vi "_PC_Daemon_TurboPump.vi"(7 "engModeStr":refnum<vi>, 8 "error in (no error)":errorcluster) -> (0 "error out":errorcluster)   [LabVIEW 2018]
uses:
  Turbo/turboState.ctl
  PublicSubVI/Ctl/RegistyFunc.ctl
  <vilib>/event_ctls.llb/eventvkey.ctl
  PublicSubVI/Class/QMH/QMH.lvclass
panel:
  out "Turbo Status":string
  in  "rotating_speed":dbl caption="rot.speed (%)"
  in  "SinpleMode.Pump On":bool
  in  "TC110 Settings":T1
  out "stop":bool
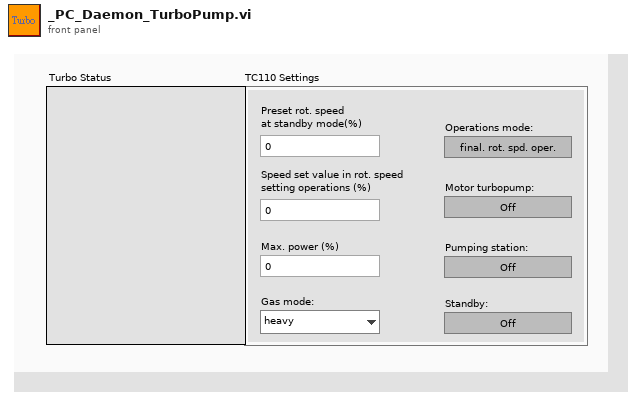
[diagram p1: front panel]
types:
  T1 = cluster{"Preset rot. speed \nat standby mode(%)":dbl, "Speed set value in rot. speed \nsetting operations (%)":dbl, "Max. power (%)":dbl, "Gas mode: ":enum16{"heavy", "light", "helium"}, "Operations mode: ":bool, "Motor turbopump: ":bool, "Pumping station: ":bool, "Standby: ":bool}
  T2 = typedef "turboState.ctl" = enum16{"setRefnum", "init", "setParam", "close"}
  T3 = cluster{"turboClusterRefnum":refnum<vi>, "pumpOnRefnum":refnum<vi>, "rotSpdRefnum":refnum<vi>}
  T4 = enum8{"Enabled", "Disabled", "Disabled and Grayed Out"}
  T5 = typedef "RegistyFunc.ctl" = enum16{"None", "FileAutoSave", "FileNoise", "FileSN", "ExeStatu", "WorkFolderPath", "MethodPath", "AVGItem", "LoopItem", "AutoRun", "BGColor", "LineColor", "LineWidth", "XGrid", "YGrid", "DeviceRefnum"}
  T6 = typedef "eventvkey.ctl" = enum16{"ASCII", "Enter", "Return", "Shift", "Ctrl", "Alt", "Cmd", "Opt", "Caps", "NumLock", "Clear", "Break", "Up", "Down", "Left", "Right", "Insert", "Delete", "Home", "End", "PageUp", "PageDown", "Escape", "Help", "Pause", "ScrollLock", "F1", "F2", "F3", "F4", "F5", "F6", "F7", "F8", "F9", "F10", "F11", "F12", "F13", "F14", "F15", "F16", "F17", "F18", "F19", "F20", "F21", "F22", "F23", "F24", "Play", "VolumeUp", "VolumeDown", "Mute", "Two Byte Char"}
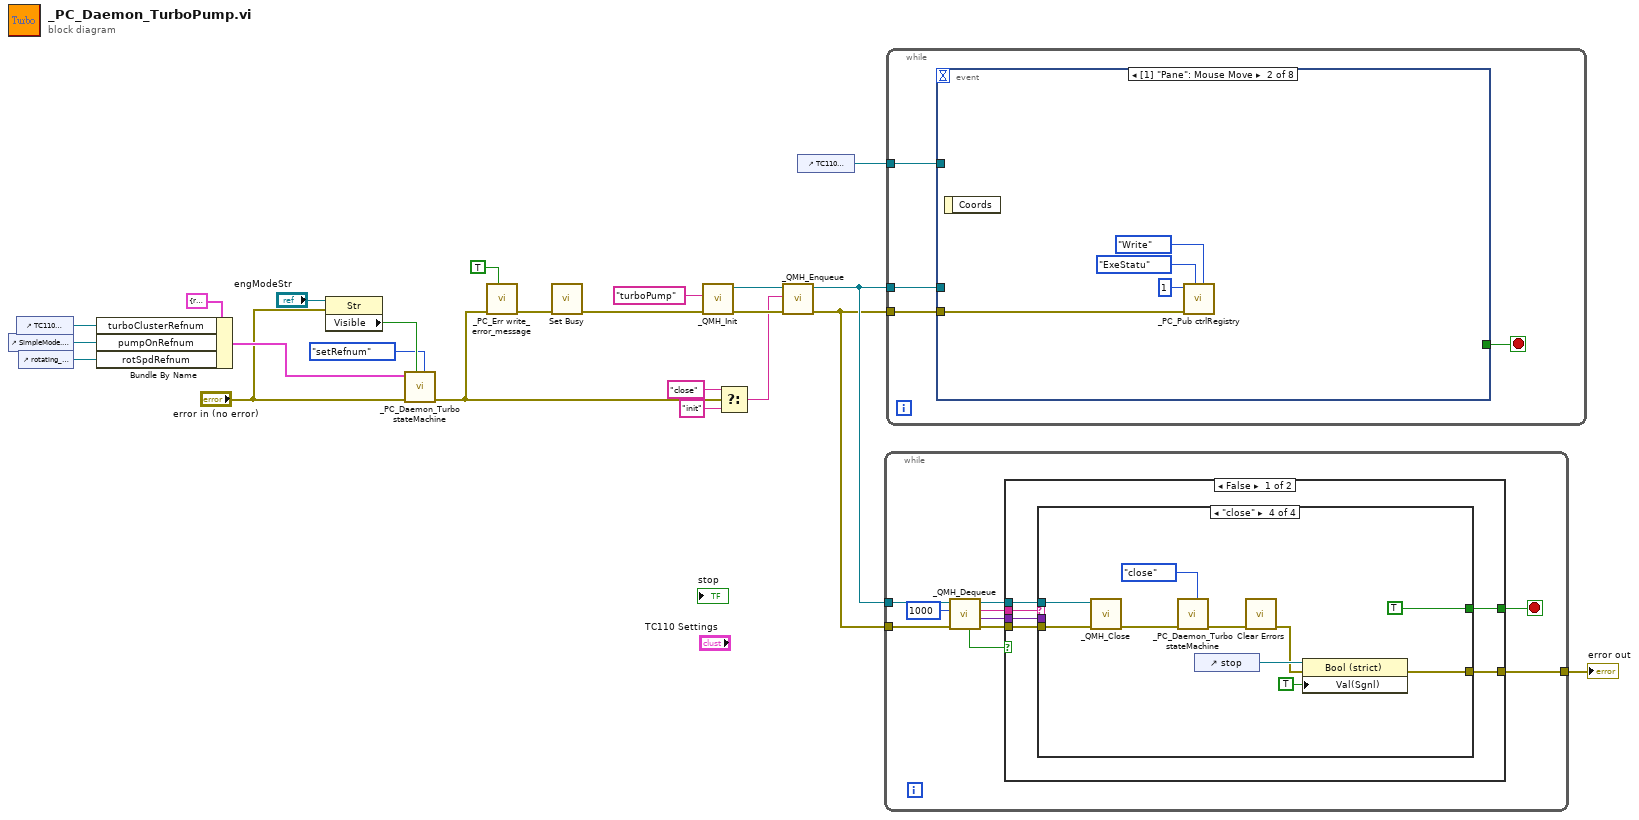
[diagram p0: block diagram]
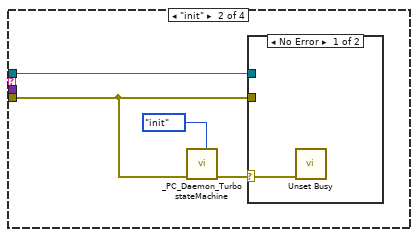
[diagram p3: hidden frame]
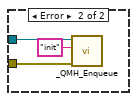
[diagram p4: hidden frame]
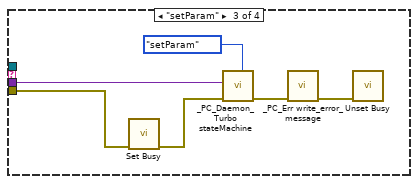
[diagram p5: hidden frame]
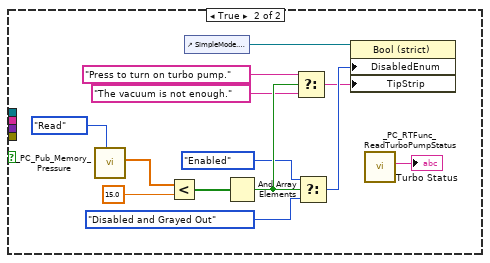
[diagram p6: hidden frame]
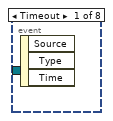
[diagram p7: hidden frame]
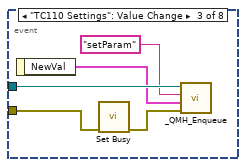
[diagram p8: hidden frame]
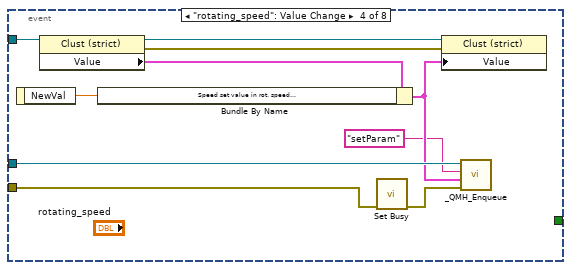
[diagram p9: hidden frame]
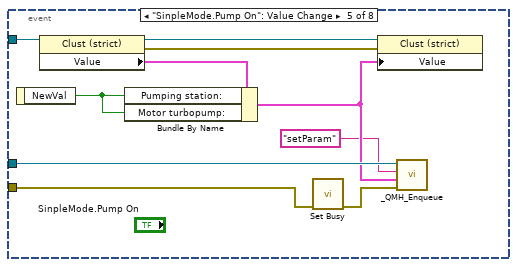
[diagram p10: hidden frame]
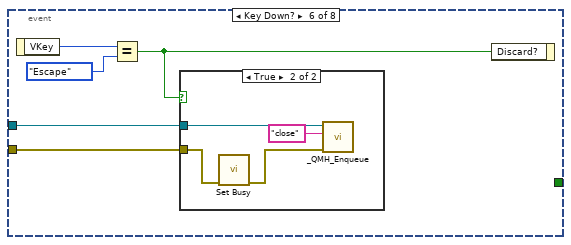
[diagram p11: hidden frame]
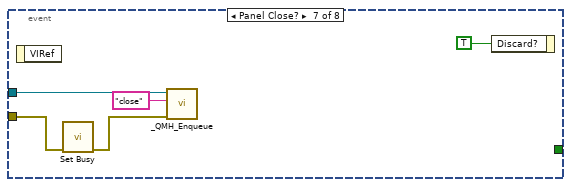
[diagram p13: hidden frame]
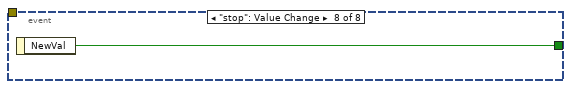
[diagram p14: hidden frame]
diagram:
  n1 = control-ref of="SimpleMode.Pump On"() -> (w10:refnum<vi>)
  n2 = control-ref of="TC110 Settings"() -> (w11:refnum<vi>)
  n3 = control-ref of="rotating_speed"() -> (w9:refnum<vi>)
  n4 = Bundle By Name(cluster=T3 {"turboClusterRefnum"=refnum, "pumpOnRefnum"=refnum, "rotSpdRefnum"=refnum} ("refnumCluster"), "turboClusterRefnum"=w11, "pumpOnRefnum"=w10, "rotSpdRefnum"=w9) -> (w15:T3)
  n5 = property class="Str"(reference="engModeStr", error in="error in (no error)") -> ("Visible"=w13:bool)  [unwired: 2 out]
  n6 = call "_PC_Daemon_Turbo stateMachine.vi"("state"=turboState."setRefnum", "engMode"=w13, "error in"="error in (no error)", "refnumCluster"=w15) -> ("error out"=w5:errorcluster)  [unwired: 7 in]
  n7 = call "_PC_Err write_error_message.vi"("show msg( T )"=TRUE, "error in"=w5) -> ("error out"=w4:errorcluster)  [unwired: 9 in]
  n8 = call <vilib>:"Set Busy.vi"("error in (no error)"=w4) -> ("error out"=w3:errorcluster)  [unwired: 9 in, 1 out]
  n9 = call "_QMH_Init.vi"("error in (no error)"=w3, "name (unnamed)"="turboPump") -> ("error out"=w21:errorcluster, "QMH out"=w22:refnum<class "QMH.lvclass">)  [unwired: 8 in]
  n10 = Select(t="close" ("Msg"), s=w5, f="init" ("Msg")) -> (s? t:f=w6:string)
  n11 = call "_QMH_Enqueue.vi"("error in (no error)"=w21, "Msg"=w6, "QMH in"=w22) -> ("error out"=w17:errorcluster, "QMH out"=w18:refnum<class "QMH.lvclass">)  [unwired: 7 in]
  n12 = control-ref of="TC110 Settings"() -> (w20:refnum<vi>)
  n13 = while {
    tunnel: w18 -> [w33]
    tunnel: w17 -> [w32]
    tunnel: [w24] -> w1
    stop <- w25 stop-if-true
    n14 = call "_QMH_Dequeue.vi"("error in (no error)"=w32, "timeout in ms (-1)"=1000, "QMH in"=w33) -> ("error out"=w28:errorcluster, "Data"=w29:variant, "Msg"=w30:string, "QMH out"=w27:refnum<class "QMH.lvclass">, "timed out?"=w26:bool)  [unwired: 3 in, 1 out]
    n15 = case shown="False" w26 {
      tunnel: w30 -> [w39 _]
      tunnel: w29 -> [w38 _]
      tunnel: w28 -> [w37 _]
      tunnel: w27 -> [w36 _]
      tunnel: [w35 _] -> w25
      tunnel: [w34 _] -> w24
      frame False {
        n16 = case shown="\"close\"" w39 {
          tunnel: w38 -> [_ _ w53 _]
          tunnel: w37 -> [_ w42 w52 w62]
          tunnel: w36 -> [_ w43 _ w63]
          tunnel: [_ _ _ TRUE] -> w35
          tunnel: [_ _ _ w54] -> w34
          frame Default {
          }
          frame "init" {
            n17 = call "_PC_Daemon_Turbo stateMachine.vi"("state"=turboState."init", "error in"=w42) -> ("error out"=w41:errorcluster)  [unwired: 9 in]
            n18 = case shown="No Error" w41 {
              selector: w41 -> [w44 _]
              tunnel: w43 -> [_ w47]
              tunnel: w42 -> [_ w45]
              frame No Error {
                n19 = call <vilib>:"Unset Busy.vi"("error in (no error)"=w44) -> ()  [unwired: 10 in, 1 out]
              }
              frame Error {
                n20 = call "_QMH_Enqueue.vi"("error in (no error)"=w45, "Msg"="init", "QMH in"=w47) -> ()  [unwired: 7 in, 2 out]
              }
            }
          }
          frame "setParam" {
            n21 = call <vilib>:"Set Busy.vi"("error in (no error)"=w52) -> ("error out"=w51:errorcluster)  [unwired: 9 in, 1 out]
            n22 = call "_PC_Daemon_Turbo stateMachine.vi"("state"=turboState."setParam", "error in"=w51, "newData"=w53) -> ("error out"=w50:errorcluster)  [unwired: 8 in]
            n23 = call "_PC_Err write_error_message.vi"("error in"=w50) -> ("error out"=w49:errorcluster)  [unwired: 10 in]
            n24 = call <vilib>:"Unset Busy.vi"("error in (no error)"=w49) -> ()  [unwired: 10 in, 1 out]
          }
          frame "close" {
            n25 = call "_QMH_Close.vi"("error in (no error)"=w62, "QMH in"=w63) -> ("error out"=w57:errorcluster)  [unwired: 9 in]
            n26 = call "_PC_Daemon_Turbo stateMachine.vi"("state"=turboState."close", "error in"=w57) -> ("error out"=w56:errorcluster)  [unwired: 9 in]
            n27 = control-ref of="stop"() -> (w59:refnum<vi>)
            n28 = call <vilib>:"Clear Errors.vi"("error in (no error)"=w56) -> ("error out"=w55:errorcluster)  [unwired: 5 in, 1 out]
            n29 = property class="Bool (strict)"(reference=w59, error in=w55, "Val(Sgnl)"=TRUE ("Value (Signaling)")) -> (error out=w54:errorcluster)  [unwired: 1 out]
          }
        }
      }
      frame True {
        n30 = call "_PC_Pub_Memory_Pressure.vi"("Function"=enum16{"Init", "Write", "Read"}."Read") -> ("Pressures"=w72:dbl[])  [unwired: 9 in, 1 out]
        n31 = Less?(x=w72, y=15.0) -> (x < y?=w73:bool[])
        n32 = control-ref of="SimpleMode.Pump On"() -> (w64:refnum<vi>)
        n33 = And Array Elements(Boolean array=w73) -> (logical AND=w76:bool)
        n34 = Select(t="Press to turn on turbo pump.", s=w76, f="The vacuum is not enough.") -> (s? t:f=w74:string)
        n35 = Select(t=T4."Enabled" ("Disabled"), s=w76, f=T4."Disabled and Grayed Out" ("Disabled")) -> (s? t:f=w75:T4)
        n36 = property class="Bool (strict)"(reference=w64, "DisabledEnum"=w75, "TipStrip"=w74) -> ()  [unwired: 1 in, 2 out]
        n37 = call "_PC_RTFunc_ReadTurboPumpStatus.vi"() -> ("TurboStatus_string"=→"Turbo Status":string)  [unwired: 8 in, 3 out]
      }
    }
  }
  "error out" <- w1
  n38 = while {
    tunnel: w17 -> [w79]
    tunnel: w18 -> [w80]
    tunnel: w20 -> [w78]
    stop <- w77 stop-if-true
    n39 = event shown="[1] \"Pane\": Mouse Move" {
      selector: _ -> [_ _ _ _ _ _ _ _]
      dyn-events: _ -> [_ _ _ _ _ _ _ _]
      timeout: _ -> [_ _ _ _ _ _ _ _]
      tunnel: w80 -> [_ _ w89 w99 w109 w111 w121 _]
      tunnel: w79 -> [_ w81 w86 w98 w108 w112 w120 _]
      tunnel: w78 -> [_ _ _ w96 w106 _ _ _]
      tunnel: [_ _ _ _ _ _ _ w124] -> w77
      event Timeout {
        n40 = event-data() -> ()  [unwired: 1 in, 3 out]
      }
      event Mouse Move {
        n41 = event-data() -> ()  [unwired: 1 in, 1 out]
        n42 = call "_PC_Pub ctrlRegistry.vi"("type"=enum16{"None", "Write", "Read"}."Write", "function"=RegistyFunc."ExeStatu", "error in (no error)"=w81, "write value"=u32 1) -> ()  [unwired: 4 in, 4 out]
      }
      event "TC110 Settings": Value Change {
        n43 = event-data() -> ("NewVal"=w87:T1)  [unwired: 1 in]
        n44 = call <vilib>:"Set Busy.vi"("error in (no error)"=w86) -> ("error out"=w85:errorcluster)  [unwired: 9 in, 1 out]
        n45 = call "_QMH_Enqueue.vi"("error in (no error)"=w85, "Data"=w87, "Msg"="setParam", "QMH in"=w89) -> ()  [unwired: 6 in, 2 out]
      }
      event "rotating_speed": Value Change {
        n46 = event-data() -> ("NewVal"=w94:dbl)  [unwired: 1 in]
        n47 = property class="Clust (strict)"(reference=w96) -> (reference out=w93:refnum<vi>, error out=w92:errorcluster, "Value"=w95:T1)  [unwired: 1 in]
        n48 = Bundle By Name(cluster=w95, "Speed set value in rot. speed \nsetting operations (%)"=w94) -> (w91:T1)
        n49 = call <vilib>:"Set Busy.vi"("error in (no error)"=w98) -> ("error out"=w97:errorcluster)  [unwired: 9 in, 1 out]
        n50 = property class="Clust (strict)"(reference=w93, error in=w92, "Value"=w91) -> ()  [unwired: 2 out]
        n51 = call "_QMH_Enqueue.vi"("error in (no error)"=w97, "Data"=w91, "Msg"="setParam", "QMH in"=w99) -> ()  [unwired: 6 in, 2 out]
      }
      event "SinpleMode.Pump On": Value Change {
        n52 = event-data() -> ("NewVal"=w100:bool)  [unwired: 1 in]
        n53 = property class="Clust (strict)"(reference=w106) -> (reference out=w104:refnum<vi>, error out=w103:errorcluster, "Value"=w105:T1)  [unwired: 1 in]
        n54 = Bundle By Name(cluster=w105, "Pumping station:"=w100, "Motor turbopump:"=w100) -> (w102:T1)
        n55 = call <vilib>:"Set Busy.vi"("error in (no error)"=w108) -> ("error out"=w107:errorcluster)  [unwired: 9 in, 1 out]
        n56 = property class="Clust (strict)"(reference=w104, error in=w103, "Value"=w102) -> ()  [unwired: 2 out]
        n57 = call "_QMH_Enqueue.vi"("error in (no error)"=w107, "Data"=w102, "Msg"="setParam", "QMH in"=w109) -> ()  [unwired: 6 in, 2 out]
      }
      event Key Down? {
        n58 = event-data() -> ("VKey"=w114:T6)  [unwired: 1 in]
        n59 = Equal?(x=w114, y=eventvkey."Escape") -> (x = y?=w110:bool)
        n60 = case shown="True" w110 {
          tunnel: w112 -> [_ w118]
          tunnel: w111 -> [_ w116]
          frame False {
          }
          frame True {
            n61 = call <vilib>:"Set Busy.vi"("error in (no error)"=w118) -> ("error out"=w117:errorcluster)  [unwired: 9 in, 1 out]
            n62 = call "_QMH_Enqueue.vi"("error in (no error)"=w117, "Msg"="close", "QMH in"=w116) -> ()  [unwired: 7 in, 2 out]
          }
        }
        n63 = event-data("Discard?"=w110) -> ()  [unwired: 1 in, 1 out]
      }
      event Panel Close? {
        n64 = event-data() -> ()  [unwired: 1 in, 1 out]
        n65 = call <vilib>:"Set Busy.vi"("error in (no error)"=w120) -> ("error out"=w123:errorcluster)  [unwired: 9 in, 1 out]
        n66 = call "_QMH_Enqueue.vi"("error in (no error)"=w123, "Msg"="close", "QMH in"=w121) -> ()  [unwired: 7 in, 2 out]
        n67 = event-data("Discard?"=TRUE) -> ()  [unwired: 1 in, 1 out]
      }
      event "stop": Value Change {
        n68 = event-data() -> ("NewVal"=w124:bool)  [unwired: 1 in]
      }
    }
  }
